vi "Less Simple Error Handler.vi"(0 "message":string, 2 "Action":enum16{"Run", "SetLevel"}(ring), 3 "error in":errorcluster, 4 "Level":u8) -> ()   [LabVIEW 2017]
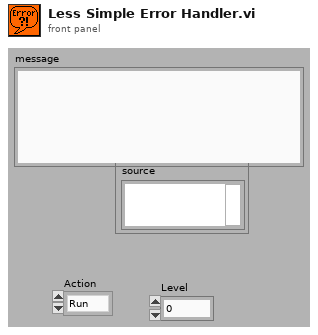
[diagram p1: front panel]
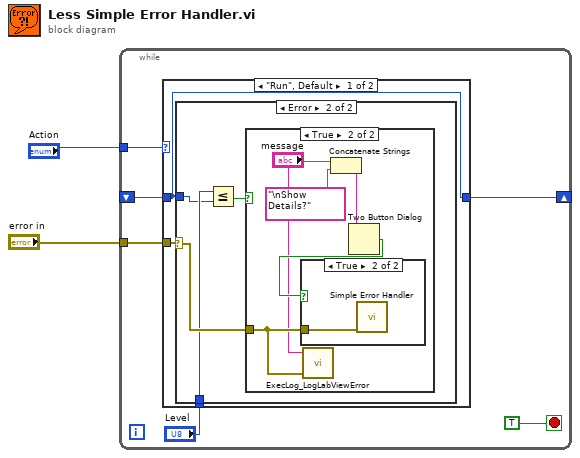
[diagram p0: block diagram]
diagram:
  n1 = while {
    tunnel: "error in" -> [w8]
    tunnel: "Action" -> [w6]
    shift-right: [w5] -> _
    shift-left: _ -> [w4]
    stop <- TRUE stop-if-true
    n2 = case shown="\"Run\", Default" w6 {
      tunnel: w8 -> [w11 _]
      tunnel: [w10 w22] -> w5
      tunnel: w4 -> [w10 _]
      tunnel: "Level" -> [w9 w22]
      frame "Run", Default {
        n3 = case shown="Error" w11 {
          selector: w11 -> [_ w15]
          tunnel: w10 -> [_ w12]
          tunnel: w9 -> [_ w14]
          frame No Error {
          }
          frame Error {
            n4 = Less Or Equal?(x=w14, y=w12) -> (x <= y?=w13:bool)
            n5 = case shown="True" w13 {
              tunnel: w15 -> [_ w17]
              frame False {
              }
              frame True {
                n6 = call "ExecLog_LogLabViewError.vi"("error IO"=w17, "string 1"="message") -> ()  [unwired: 1 in]
                n7 = Concatenate Strings("message", "\nShow Details?" ("string")) -> (w18:string)
                n8 = Two Button Dialog(message=w18) -> (T button?=w20:bool)  [unwired: 2 out]
                n9 = case shown="True" w20 {
                  tunnel: w17 -> [_ w21]
                  frame False {
                  }
                  frame True {
                    n10 = call <vilib>:"Simple Error Handler.vi"("error in (no error)"=w21) -> ()  [unwired: 1 in, 8 out]
                  }
                }
              }
            }
          }
        }
      }
      frame "SetLevel" {
      }
    }
  }
